vi "Encoder_Initialization(SubVI).vi"(8 "error in (no error)":errorcluster, 11 "refnum":T2) -> (0 "error out":errorcluster, 2 "Encoder values":T1, 3 "refnum out":T2)   [LabVIEW 2017]
uses:
  <vilib>/Utility/config.llb/Config Data RefNum.ctl
  <vilib>/Utility/config.llb/Read Key (Double).vi
  <vilib>/Utility/config.llb/NI_LVConfig.lvlib
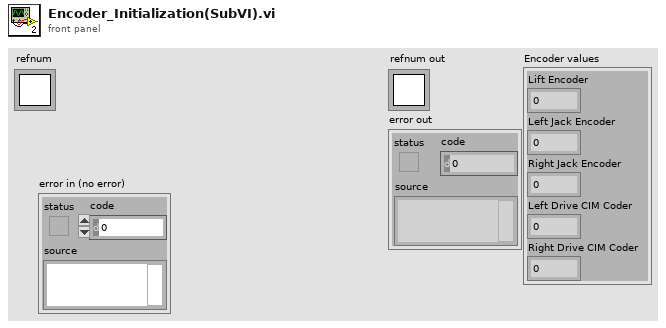
[diagram p1: front panel]
types:
  T1 = cluster{"Lift Encoder":dbl, "Left Jack Encoder":dbl, "Right Jack Encoder":dbl, "Left Drive CIM Coder":dbl, "Right Drive CIM Coder":dbl}
  T2 = typedef "NI_LVConfig.lvlib/Config Data RefNum.ctl" = refnum<k1>
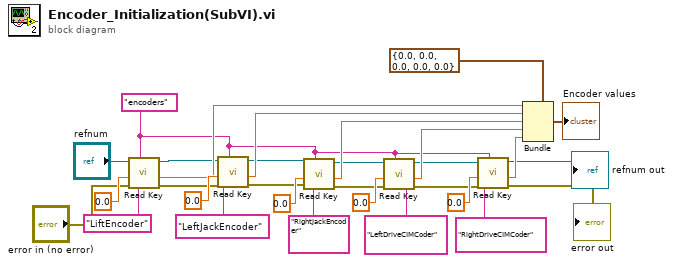
[diagram p0: block diagram]
diagram:
  w1 = "encoders" ("section")
  n1 = call-poly <vilib>:"Read Key.vi"("section"=w1, "error in (no error)"="error in (no error)", "default value"=0.0, "key"="LiftEncoder", "refnum"="refnum") -> ("error out"=w11:errorcluster, "value"=w21:dbl, "refnum out"=w7:T2)  [unwired: 3 in, 1 out]
  n2 = call-poly <vilib>:"Read Key.vi"("section"=w1, "error in (no error)"=w11, "default value"=0.0, "key"="LeftJackEncoder", "refnum"=w7) -> ("error out"=w12:errorcluster, "value"=w22:dbl, "refnum out"=w8:T2)  [unwired: 3 in, 1 out]
  n3 = call-poly <vilib>:"Read Key.vi"("section"=w1, "error in (no error)"=w12, "default value"=0.0, "key"="RightJackEncoder", "refnum"=w8) -> ("error out"=w13:errorcluster, "value"=w23:dbl, "refnum out"=w9:T2)  [unwired: 3 in, 1 out]
  n4 = call-poly <vilib>:"Read Key.vi"("section"=w1, "error in (no error)"=w13, "default value"=0.0, "key"="LeftDriveCIMCoder", "refnum"=w9) -> ("error out"=w14:errorcluster, "value"=w24:dbl, "refnum out"=w10:T2)  [unwired: 3 in, 1 out]
  n5 = call-poly <vilib>:"Read Key.vi"("section"=w1, "error in (no error)"=w14, "default value"=0.0, "key"="RightDriveCIMCoder", "refnum"=w10) -> ("error out"=→"error out":errorcluster, "value"=w25:dbl, "refnum out"=→"refnum out":T2)  [unwired: 3 in, 1 out]
  n6 = Bundle(cluster=T1 {"Lift Encoder"=0.0, "Left Jack Encoder"=0.0, "Right Jack Encoder"=0.0, "Left Drive CIM Coder"=0.0, "Right Drive CIM Coder"=0.0} ("Encoder values"), "Lift Encoder"=w21, "Left Jack Encoder"=w22, "Right Jack Encoder"=w23, "Left Drive CIM Coder"=w24, "Right Drive CIM Coder"=w25) -> (→"Encoder values":T1)
